vi "Compensate Gain.vi"(0 "i":fxp<+/-,18,1>, 1 "reset":bool, 5 "q":fxp<+/-,37,3>, 7 "gain":fxp<+/-,18,3>, 9 "input valid":bool) -> (4 "iq data":T1, 10 "output valid":bool)   [LabVIEW 2017, in "NI PLL IP FPGA.lvlib"]
uses:
  NI PLL IP FPGA.lvlib
  <instrlib>/_niInstr/DSP/v1/Shared/Public/IQ Data.ctl
  <vilib>/rvi/FXPMathLib/FxpMul/XNode/nifxpmath_Multiplier.xnode
  <instrlib>/_niInstr/DSP/v1/Shared/niInstr DSP v1 Shared.lvlib
  <vilib>/rvi/FXPMathLib/sim/FxpSim.dll
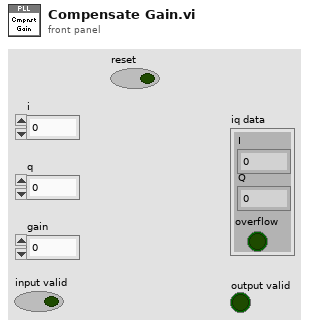
[diagram p1: front panel]
types:
  T1 = typedef "niInstr DSP v1 Shared.lvlib/IQ Data.ctl" = cluster{"I":fxp<+/-,18,1>, "Q":fxp<+/-,18,1>, "overflow":bool}
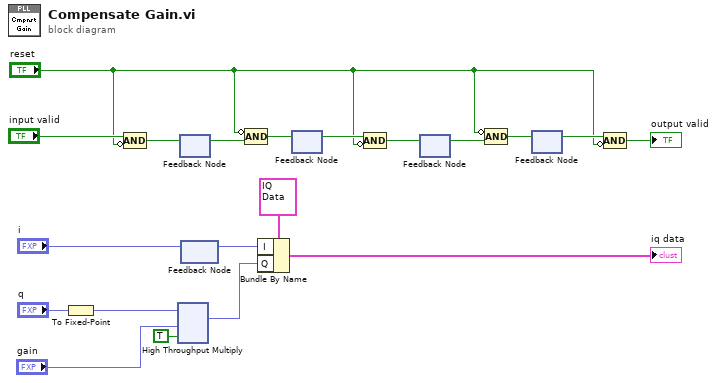
[diagram p0: block diagram]
diagram:
  n1 = To Fixed-Point(number="q") -> (fixed-point=w18:fxp<+/-,25,3>)  [unwired: 1 in]
  n2 = Compound Arithmetic op=AND("input valid", invert "reset") -> (w9:bool)
  n3 = xnode "High Throughput Multiply"("x"=w18, "y"="gain", "input valid"=TRUE) -> ("x*y"=w14:fxp<+/-,18,1>)  [unwired: 1 in, 2 out]
  n4 = feedback #1() -> (w11:bool)  [unwired: 1 in]
  n5 = feedback-in #1(w9) -> ()
  n6 = feedback-in #2("i") -> ()
  n7 = feedback #2() -> (w16:fxp<+/-,18,1>)  [unwired: 1 in]
  n8 = Compound Arithmetic op=AND(invert "reset", w11) -> (w8:bool)
  n9 = Bundle By Name(cluster=T1 {"I"=0.0, "Q"=0.0, "overflow"=FALSE} ("data"), "I"=w16, "Q"=w14) -> (→"iq data":T1)
  n10 = feedback #3() -> (w7:bool)  [unwired: 1 in]
  n11 = feedback-in #3(w8) -> ()
  n12 = Compound Arithmetic op=AND(w7, invert "reset") -> (w3:bool)
  n13 = feedback #4() -> (w4:bool)  [unwired: 1 in]
  n14 = feedback-in #4(w3) -> ()
  n15 = Compound Arithmetic op=AND(invert "reset", w4) -> (w5:bool)
  n16 = feedback #5() -> (w6:bool)  [unwired: 1 in]
  n17 = feedback-in #5(w5) -> ()
  n18 = Compound Arithmetic op=AND(w6, invert "reset") -> (→"output valid":bool)
